vi "SR_CORE.vi"(8 "错误输入（无错误）":errorcluster, 10 "phrases":string[](array[string]), 11 "SR_REC_TEXT":refnum<vi>) -> (0 "错误输出":errorcluster caption="error out", 3 ".NET引用句柄输出":refnum<k24>)   [LabVIEW 2018]
uses:
  System.Speech
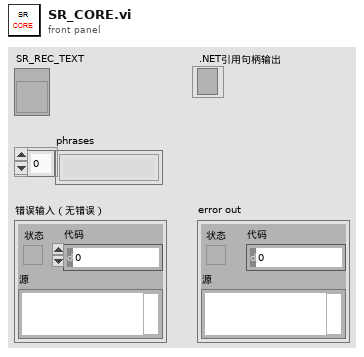
[diagram p1: front panel]
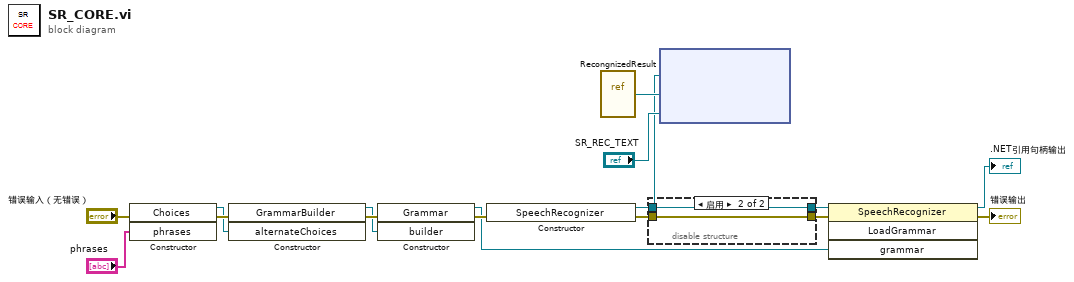
[diagram p0: block diagram]
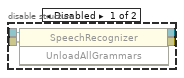
[diagram p2: hidden frame]
diagram:
  n1 = constructor class="Choices"(error in="错误输入（无错误）", "phrases"="phrases") -> (reference out=w2:refnum<k24>, error out=w6:errorcluster)  [unwired: 2 in, 2 out]
  n2 = constructor class="GrammarBuilder"(error in=w6, "alternateChoices"=w2) -> (reference out=w4:refnum<k24>, error out=w9:errorcluster)  [unwired: 2 in, 2 out]
  n3 = constructor class="Grammar"(error in=w9, "builder"=w4) -> (reference out=w5:refnum<k24>, error out=w10:errorcluster)  [unwired: 2 in, 2 out]
  n4 = constructor class="SpeechRecognizer"(error in=w10) -> (reference out=w13:refnum<k24>, error out=w7:errorcluster)  [unwired: 2 in, 1 out]
  n5 = vi-ref "RecongnizedResult.vi"() -> (w15:refnum<vi>)
  n6 = disable-structure shown="启用" {
    disable-tunnel: w13 -> [w20 w22]
    disable-tunnel: [w19 w21] -> w8
    disable-tunnel: w7 -> [w18 w21]
    disable-tunnel: [w17 w22] -> w3
    frame Disabled {
      n7 = invoke class="SpeechRecognizer" method="UnloadAllGrammars"(reference=w20, error in=w18) -> (reference out=w17:refnum<k24>, error out=w19:errorcluster)  [unwired: 1 in, 1 out]
    }
    frame Enabled {
    }
  }
  n8 = node(w13, w15, "SR_REC_TEXT") -> ()  [unwired: 2 in, 2 out]
  n9 = invoke class="SpeechRecognizer" method="LoadGrammar"(reference=w3, error in=w8, "grammar"=w5) -> (reference out=→".NET引用句柄输出":refnum<k24>, error out=→"错误输出":errorcluster)  [unwired: 1 in, 2 out]
